vi "ModifyAttribute.vi"(0 "reference in":refnum<class "G#BaseClass2.lvclass">, 1 "Lock time (ms)":u32, 2 "timeout in ms (-1)":i32=-1, 3 "Unlock data if error? (T)":bool=TRUE, 4 "Only unlock data? (F)":bool, 5 "error in (no error)":errorcluster, 7 "status":bool) -> (14 "reference out":refnum<class "G#BaseClass2.lvclass">, 16 "timeout":bool, 19 "error out":errorcluster)   [LabVIEW 2020, in "G#BaseClass2.lvclass"]
uses:
  G#BaseClass2.lvclass
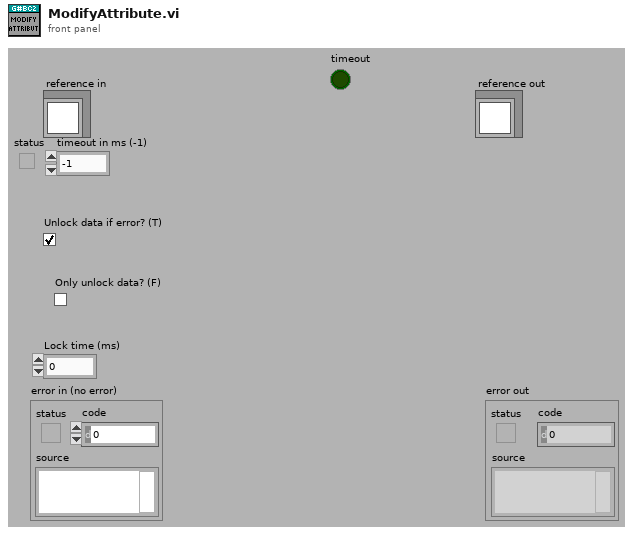
[diagram p1: front panel]
types:
  T1 = typedef "G#BaseClass2.lvclass/ObjectAttributes.ctl" = cluster{"Numeric":dbl, "Array":dbl[]}
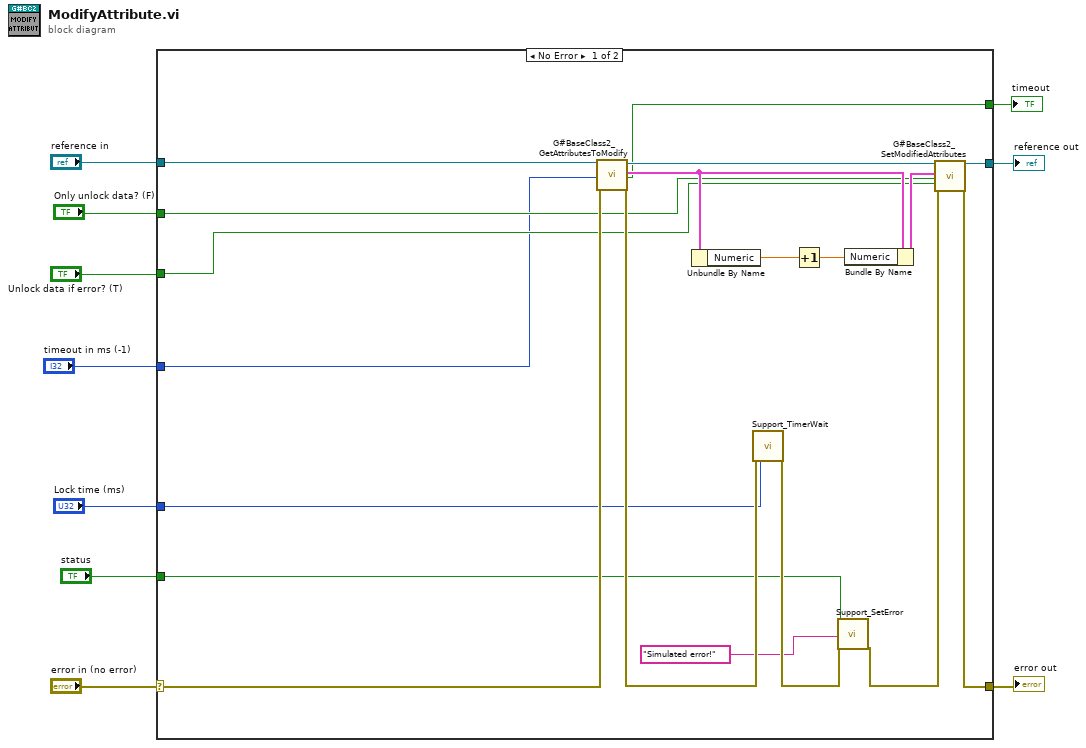
[diagram p0: block diagram]
diagram:
  n1 = case shown="No Error" "error in (no error)" {
    selector: "error in (no error)" -> [w25 w31]
    tunnel: [w27 w31] -> w9
    tunnel: [w24 w30] -> w7
    tunnel: "reference in" -> [w26 w30]
    tunnel: "Lock time (ms)" -> [w19 _]
    tunnel: "Only unlock data? (F)" -> [w18 _]
    tunnel: "Unlock data if error? (T)" -> [w17 _]
    tunnel: "status" -> [w13 _]
    tunnel: [w12 _] -> w2
    tunnel: "timeout in ms (-1)" -> [w11 _]
    frame No Error {
      n2 = call "G#BaseClass2_GetAttributesToModify.vi"("reference in"=w26, "timeout in ms (-1)"=w11, "error in (no error)"=w25) -> ("reference out"=w28:refnum<class "G#BaseClass2.lvclass">, "attributes"=w23:T1, "timeout"=w12:bool, "error out"=w20:errorcluster)  [unwired: 12 in, 1 out]
      n3 = Unbundle By Name(w23) -> ("Numeric"=w22:dbl)
      n4 = call "Support_TimerWait.vi"("error in (no error)"=w20, "milliseconds to wait"=w19) -> ("error out"=w16:errorcluster)  [unwired: 17 in]
      n5 = Increment(x=w22) -> (x+1=w21:dbl)
      n6 = call "Support_SetError.vi"("status"=w13, "source"="Simulated error!", "error in (no error)"=w16) -> ("error out"=w15:errorcluster)  [unwired: 16 in]
      n7 = Bundle By Name(cluster=w23, "Numeric"=w21) -> (w29:T1)
      n8 = call "G#BaseClass2_SetModifiedAttributes.vi"("reference in"=w28, "attributes"=w29, "Only unlock data? (F)"=w18, "Unlock data if error? (T)"=w17, "error in (no error)"=w15) -> ("reference out"=w24:refnum<class "G#BaseClass2.lvclass">, "error out"=w27:errorcluster)  [unwired: 13 in]
    }
    frame Error {
    }
  }
  "error out" <- w9
  "reference out" <- w7
  "timeout" <- w2
